vi "Replace TAB,CR,LF by SPACE.vi"(2 "String":string) -> (7 "String with replacements":string)   [LabVIEW 2021, in "Strings.lvlib"]
uses:
  Strings.lvlib
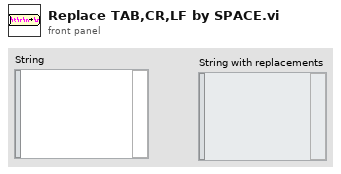
[diagram p1: front panel]
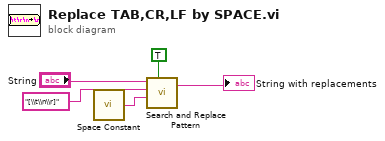
[diagram p0: block diagram]
diagram:
  n1 = call <vilib>:"Space Constant.vi"() -> ("String"=w3:string)
  n2 = call <vilib>:"Search and Replace Pattern.vi"("string"="String", "regular expression (\"\")"="[\\t\\n\\r]" ("regular expression (\"\")"), "replace string (\"\")"=w3, "replace all? (F)"=TRUE) -> ("result string"=→"String with replacements":string)  [unwired: 1 in, 1 out]
